vi "SIGLENT_SPD3303X-E_front_panel_formatka.vi"() -> ()   [LabVIEW 2020]
uses:
  controls/States_of_machine.ctl
panel:
  in  "CURR":dbl(knob) scale=0.0..3.2
  in  "Tab Control":enum32{"CH1", "CH2", "SETTINGS"}(tab)
  in  "ON/OFF CH1":bool
  out "I CH1":dbl
  out "V CH1":dbl
  out "Waveform Chart":dbl(graph)
  out "V MAX CH1":dbl
  out "I MAX CH1":dbl
  in  "ON/OFF CH2":bool
  out "Waveform Chart 2":dbl(graph)
  out "I MAX CH2":dbl
  out "V MAX CH2":dbl
  out "V CH2":dbl
  out "I CH2":dbl
  in  "stop":bool
  in  "VOLT":dbl(knob) scale=0.0..32.0
  in  "POWER":bool
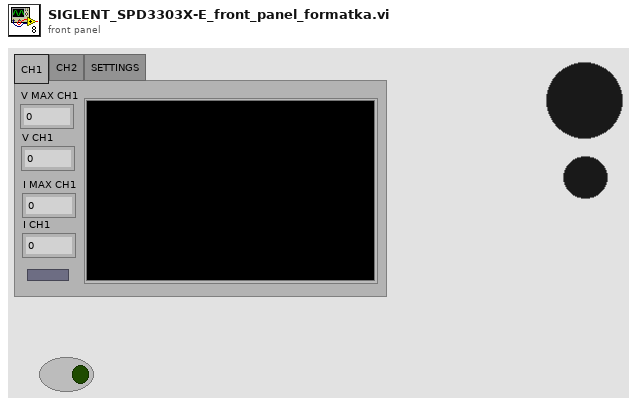
[diagram p1: front panel]
types:
  T1 = typedef "States_of_machine.ctl" = enum16{"Init", "IDLE", ""}
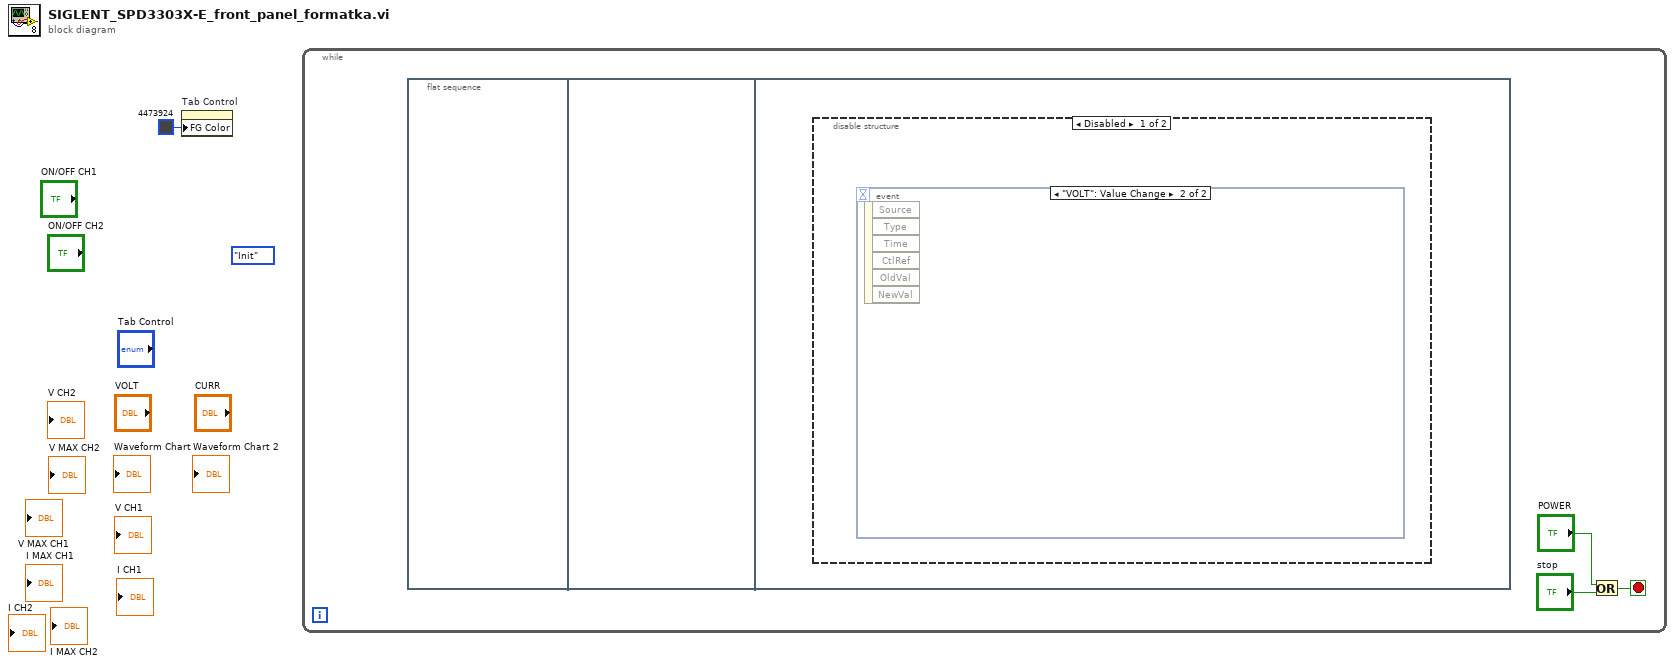
[diagram p0: block diagram]
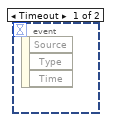
[diagram p2: hidden frame]
diagram:
  (unwired) States_of_machine."Init" ("Enum")
  n1 = property on="Tab Control" class="TabCtl (strict)"("FG Color"=u32 4473924 ("Colors:FG Color")) -> ()  [unwired: 2 in, 2 out]
  n2 = while {
    stop <- w4 stop-if-true
    n3 = flat-sequence {
      frame #0 {
      }
      frame #1 {
      }
      frame #2 {
        n4 = disable-structure shown="Disabled" {
          frame Disabled {
            n5 = event shown="[1] \"VOLT\": Value Change" {
              selector: _ -> [_ _]
              dyn-events: _ -> [_ _]
              timeout: _ -> [_ _]
              event Timeout {
                n6 = event-data() -> ()  [unwired: 1 in, 3 out]
              }
              event "VOLT": Value Change {
                n7 = event-data() -> ()  [unwired: 1 in, 6 out]
              }
            }
          }
          frame Enabled {
          }
        }
      }
    }
    n8 = Or(x="POWER", y="stop") -> (x .or. y?=w4:bool)
  }
